vi "UTIL EMG Filter_v2.vi"(8 "init/cont (init:F)":bool, 10 "Preamp Gain":dbl(ring) items=["10X"=10.0, "100X"=100.0], 11 "EMG In":waveform(dbl)) -> (1 "EMG Power":dbl format="%0.2f", 3 "Filtered EMG Out":waveform(dbl))   [LabVIEW 2010]
doc: "This VI applies a BandPass Butterworth filter to the input EMG Waveform using predetermined filter coefficients from MATLAB. It returns the Filtered EMG (80-100Hz) and the 1-s power r.m.s. power in the 80-100Hz band A notch filter at 60 Hz is also applied prior to the band filters.\n\nInputs:\n EMG In Waveform\n Preamp Gain DBL\n Init/Cont Boolean\nOutputs:\n Filtered EMG Out Waveform\n EMG Power DBL\n Error Out"
uses:
  <vilib>/Analysis/3filter.llb/IIR Filter (DBL).vi
  <vilib>/Analysis/NI_AALBase.lvlib
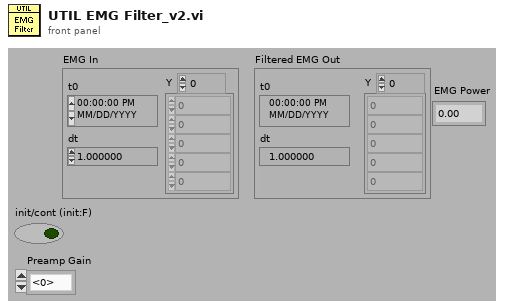
[diagram p1: front panel]
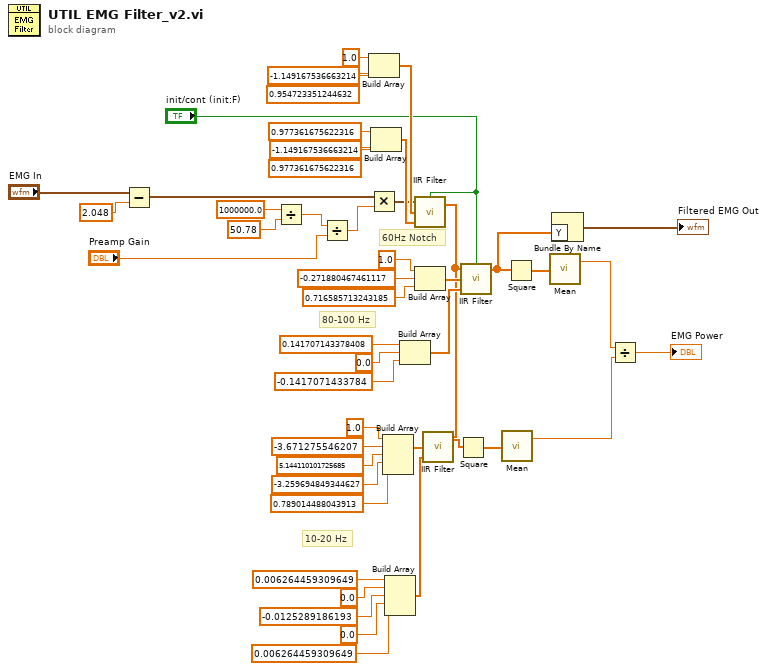
[diagram p0: block diagram]
diagram:
  # "10-20 Hz"
  # "80-100 Hz"
  # "60Hz Notch"
  n1 = Subtract(x="EMG In", y=2.048) -> (x-y=w25:waveform(dbl))
  n2 = Divide(x=1000000.0, y=50.78) -> (x/y=w21:dbl)
  n3 = Divide(x=w21, y="Preamp Gain") -> (x/y=w19:dbl)
  n4 = Build Array(1.0 ("element"), -1.149167536663214 ("element"), 0.954723351244632 ("element")) -> (w40:dbl[])
  n5 = Multiply(x=w25, y=w19) -> (x*y=w27:waveform(dbl))
  n6 = Build Array(0.977361675622316 ("element"), -1.149167536663214 ("element"), 0.977361675622316 ("element")) -> (w39:dbl[])
  n7 = Build Array(1.0 ("element"), -3.671275546207 ("element"), 5.144110101725685 ("element"), -3.259694849344627 ("element"), 0.789014488043913 ("element")) -> (w17:dbl[])
  n8 = Build Array(0.006264459309649 ("element"), 0.0 ("element"), -0.0125289186193 ("element"), 0.0 ("element"), 0.006264459309649 ("element")) -> (w18:dbl[])
  n9 = Build Array(0.141707143378408 ("element"), 0.0 ("element"), -0.1417071433784 ("element")) -> (w30:dbl[])
  n10 = call-poly <vilib>:"IIR Filter.vi"("init/cont (init:F)"="init/cont (init:F)", "Forward Coefficients"=w39, "Reverse Coefficients"=w40, "X"=w27) -> ("Filtered X"=w1:dbl[])  [unwired: 1 out]
  n11 = Build Array(1.0 ("element"), -0.271880467461117 ("element"), 0.716585713243185 ("element")) -> (w31:dbl[])
  n12 = call-poly <vilib>:"IIR Filter.vi"("Forward Coefficients"=w18, "Reverse Coefficients"=w17, "X"=w1) -> ("Filtered X"=w5:dbl[])  [unwired: 1 in, 1 out]
  n13 = Square(x=w5) -> (x^2=w6:dbl[])
  n14 = call-poly <vilib>:"IIR Filter.vi"("init/cont (init:F)"="init/cont (init:F)", "Forward Coefficients"=w30, "Reverse Coefficients"=w31, "X"=w1) -> ("Filtered X"=w29:dbl[])  [unwired: 1 out]
  n15 = call <vilib>:"Mean.vi"("X"=w6) -> ("mean"=w3:dbl)  [unwired: 1 out]
  n16 = Square(x=w29) -> (x^2=w47:dbl[])
  n17 = call <vilib>:"Mean.vi"("X"=w47) -> ("mean"=w4:dbl)  [unwired: 1 out]
  n18 = Bundle By Name("Y"=w29) -> (→"Filtered EMG Out":waveform(dbl))  [unwired: 1 in]
  n19 = Divide(x=w4, y=w3) -> (x/y=→"EMG Power":dbl)
